vi "newDataEvent.vi"(8 "error in (no error)":errorcluster, 10 "data":variant, 11 "FringeTestingViewer in":refnum<class "FringeTestingViewer.lvclass">) -> (0 "error out":errorcluster, 3 "FringeTestingViewer out":refnum<class "FringeTestingViewer.lvclass">)   [LabVIEW 2009, in "Views.lvlib" / "Camera.lvlib" / "FringeTestingViewer.lvclass"]
uses:
  FringeTestingViewer.lvclass
  FringeTestingViewer.lvclass/FringeTestingViewer.ctl
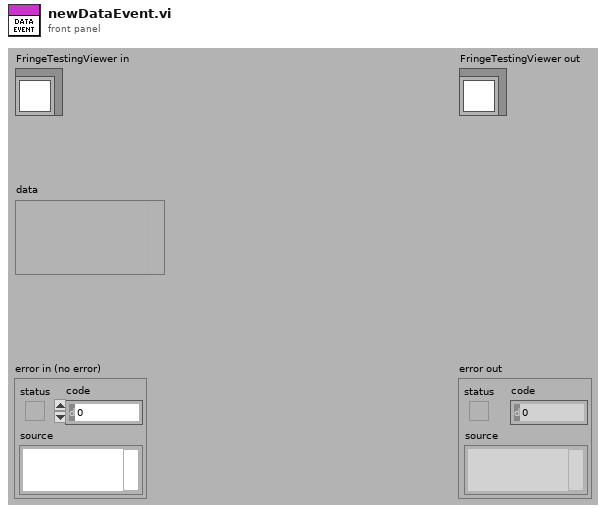
[diagram p1: front panel]
types:
  T1 = cluster{"Name":string, "Results":dbl[], "AnalysisType":string}
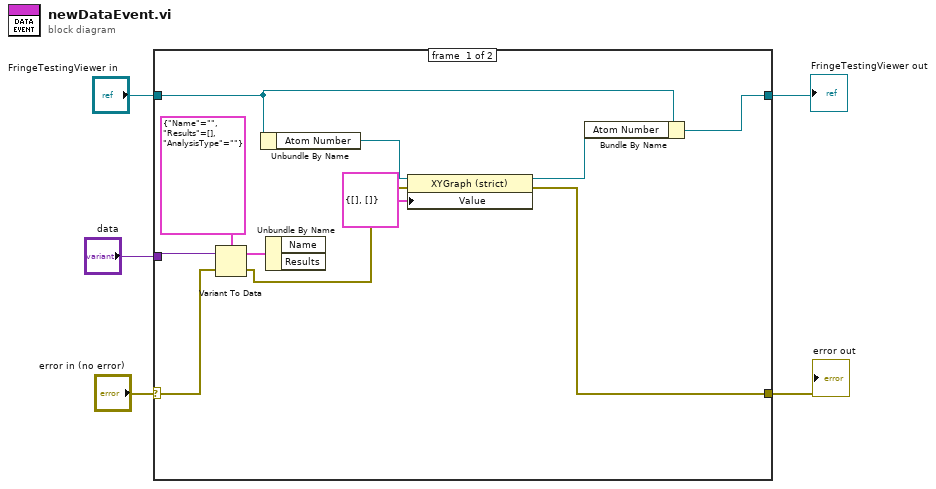
[diagram p0: block diagram]
diagram:
  n1 = case shown="No Error" "error in (no error)" {
    selector: "error in (no error)" -> [w14 w18]
    tunnel: [w7 w18] -> w4
    tunnel: [w8 w17] -> w3
    tunnel: "FringeTestingViewer in" -> [w9 w17]
    tunnel: "data" -> [w16 _]
    frame #0 {
      n2 = Variant To Data(error in=w14, Variant=w16, type=T1 {"Name"="", "Results"=[], "AnalysisType"=""} ("output cluster")) -> (error out=w11:errorcluster, data=w13:T1)
      n3 = Unbundle By Name(w9) -> ("Atom Number"=w12:refnum<vi>)
      n4 = Unbundle By Name(w13) -> ()  [unwired: 2 out]
      n5 = property class="XYGraph (strict)"(reference=w12, error in=w11, "Value"=cluster{dbl[], dbl[]} {[], []}) -> (reference out=w10:refnum<vi>, error out=w7:errorcluster)
      n6 = Bundle By Name(cluster=w9, "Atom Number"=w10) -> (w8:refnum<class "FringeTestingViewer.lvclass">)
    }
    frame #1 {
    }
  }
  "error out" <- w4
  "FringeTestingViewer out" <- w3
